vi "Gif.CommentExtension.vi"(0 "data":string, 9 "offset":i32, 11 "error in (no error)":errorcluster) -> (4 "data out":string, 6 "Comment":string, 10 "offset out":i32, 15 "error out":errorcluster)   [LabVIEW 2011]
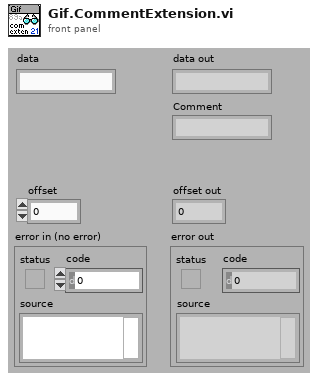
[diagram p1: front panel]
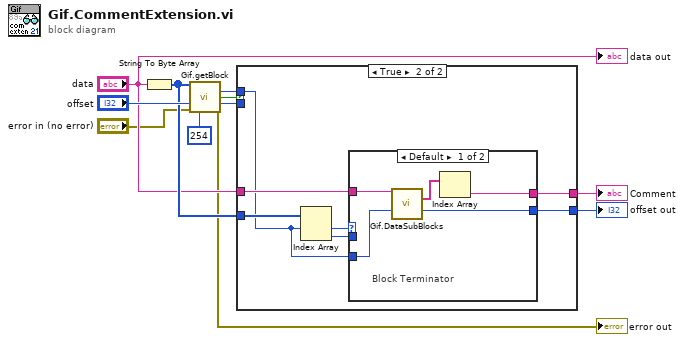
[diagram p0: block diagram]
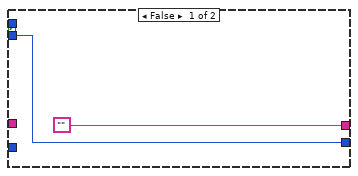
[diagram p2: hidden frame]
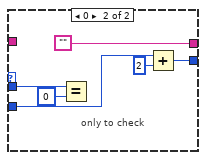
[diagram p3: hidden frame]
diagram:
  n1 = String To Byte Array(string="data") -> (unsigned byte array=w7:u8[])
  n2 = call "Gif.getBlock.vi"("data"=w7, "offset"="offset", "error in (no error)"="error in (no error)", "label"=u8 254 ("element")) -> ("pos offset"=w9:i32, "found?"=w10:bool, "offset out"=w6:i32, "error out"=→"error out":errorcluster)  [unwired: 8 out]
  n3 = case shown="True" w10 {
    tunnel: w9 -> [_ w15]
    tunnel: "data" -> [_ w18]
    tunnel: ["" w14] -> w8
    tunnel: w7 -> [_ w20]
    tunnel: w6 -> [w13 _]
    tunnel: [w13 w16] -> w5
    frame False {
    }
    frame True {
      n4 = Index Array(array=w20, index #1=w15) -> (element #1=w19:u8, element #2=w17:u8)  [unwired: 1 in]
      n5 = case shown="Default" w19 {
        tunnel: w18 -> [w25 _]
        tunnel: w15 -> [w24 w29]
        tunnel: w17 -> [_ w31]
        tunnel: [w23 w27] -> w16
        tunnel: [w21 ""] -> w14
        frame Default {
          # "Block Terminator"
          n6 = call "Gif.DataSubBlocks.vi"("data"=w25, "offset"=w24) -> ("SubBlock values"=w22:string[], "offset out"=w23:i32)  [unwired: 1 in, 11 out]
          n7 = Index Array(array=w22) -> (element=w21:string)  [unwired: 1 in]
        }
        frame 0 {
          # "only to check"
          n8 = Equal?(x=w31, y=u8 0 ("element")) -> ()  [unwired: 1 out]
          n9 = Add(x=w29, y=2) -> (x+y=w27:i32)
        }
      }
    }
  }
  "Comment" <- w8
  "offset out" <- w5
  "data out" <- "data"
